vi "CSM Batch Format Tool.vi"() -> ()   [LabVIEW 2017]
doc: "Switch the language of CSM module VI descriptions and comments. Currently supports Chinese and English."
uses:
  <vilib>/Utility/miscctls.llb/LVRectTypeDef.ctl
  _csmHelper/Utility/Is CSM Module - VIRef.vi
  _csmHelper/API/Create From Basic Refs.vi
  _csmHelper/API/Save Instrument.vi
  _csmHelper/API/Destroy.vi
  _csmDoc/csmdoc.lvlib
  Communicable State Machine.lvlib
  _csmHelper/Utility/CSM-Helper Utility.lvlib
  _csmHelper/CSM-Helper.lvclass
  _csmHelper/API/Open Front Panel.vi
panel:
  in  "Open":bool
  in  "CSM Only?":bool
  in  "Terminate":bool
  in  "Refresh":bool
  in  "Macro: Update VI Title":bool
  in  "Macro: Relocate VI Window":bool
  in  "Macro: Rename Year of copyright":bool
  out "Listbox":i32(listbox)
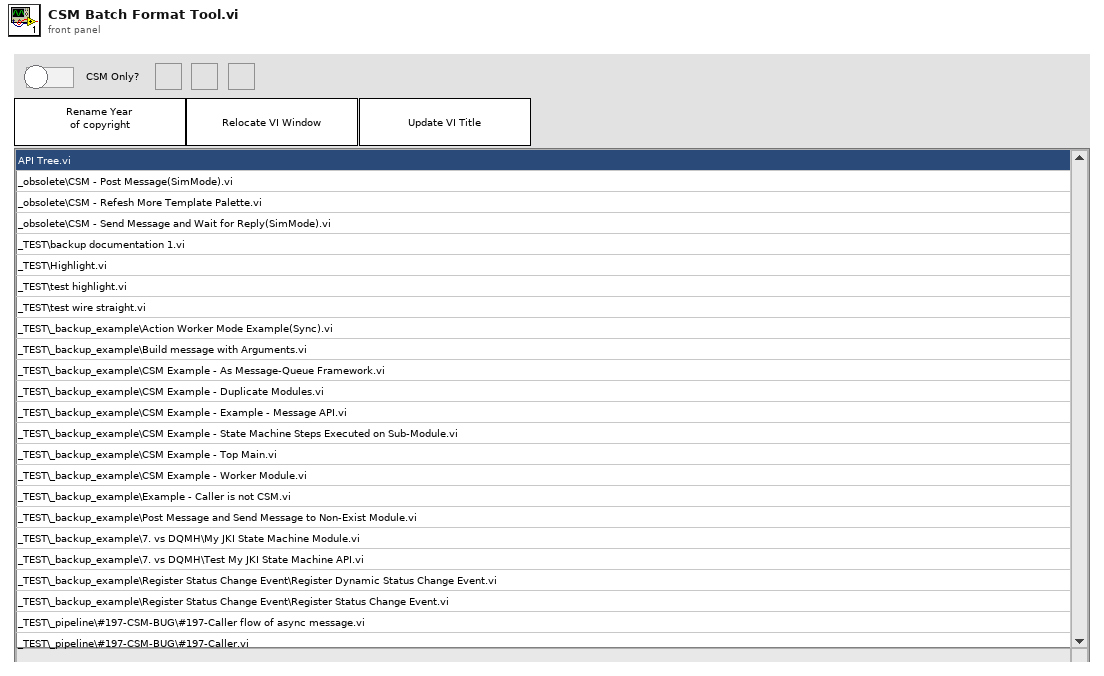
[diagram p1: front panel]
types:
  T1 = enum32{"Invalid", "Standard", "Closed", "Hidden", "Minimized", "Maximized"}
  T2 = enum32{"invalid app kind", "Development System", "Run Time System", "Student Edition", "Embedded LabVIEW", "Evaluation", "Custom"}
  T3 = cluster{"Core":cluster{"Current VI Reference":refnum<vi>, "Close Panel on Exit?":bool}, "VIs":path[], "Success":bool, "Root":path}
  T4 = cluster{"Current VI Reference":refnum<vi>, "Close Panel on Exit?":bool}
  T5 = typedef "CSM-Helper Utility.lvlib/CSM Basic Refs.ctl" = cluster{"VI":refnum<vi>, "While Loop":refnum<vi>, "Case Structure":refnum<vi>, "Parse State Queue":refnum<vi>, "Event Structure":refnum<vi>, "Type":T6}
  T6 = typedef "CSM-Helper Utility.lvlib/CSM Module Type.ctl" = enum16{"Not a CSM", "JKISM", "CSM"}
  T7 = typedef "LVRectTypeDef.ctl" = cluster{"Left":i16, "Top":i16, "Right":i16, "Bottom":i16}
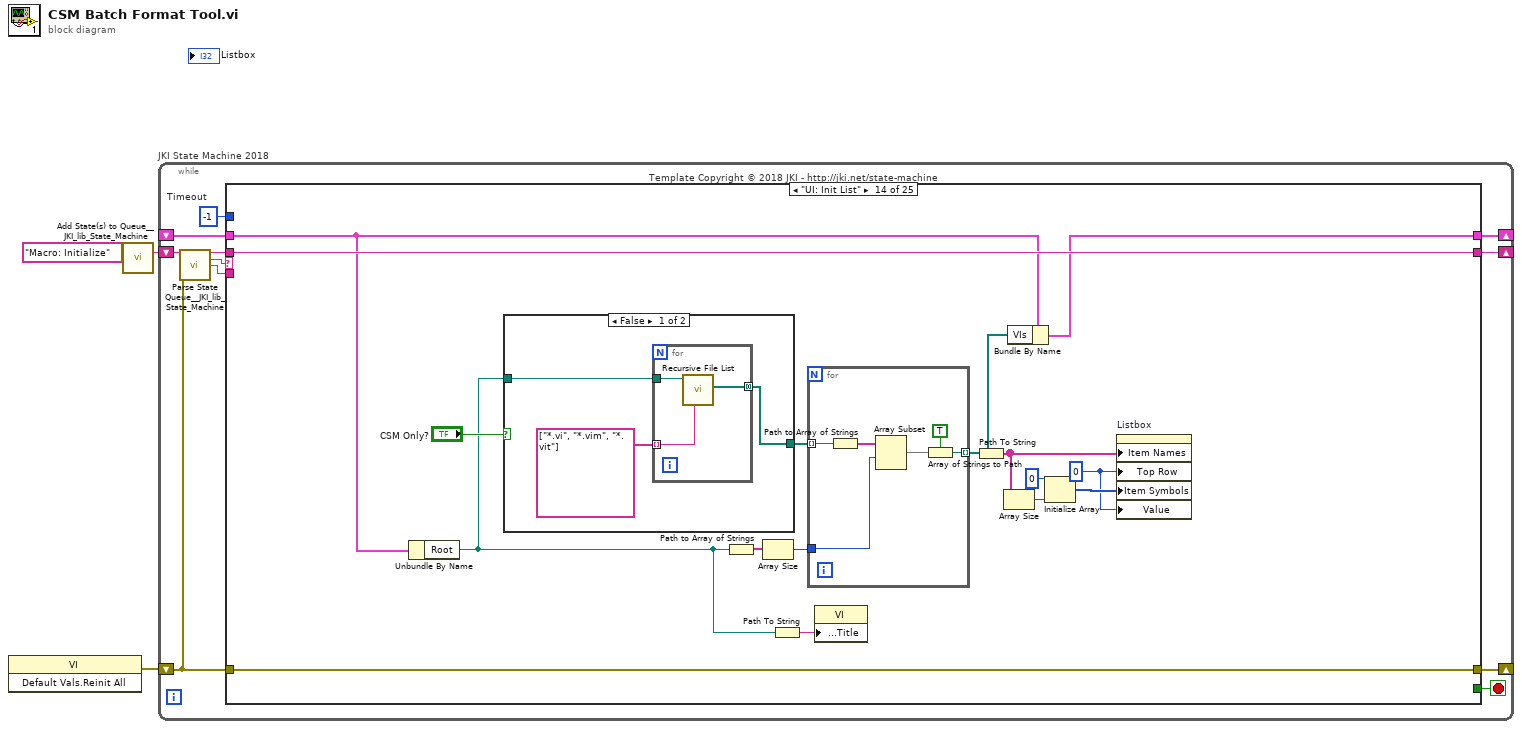
[diagram p0: block diagram]
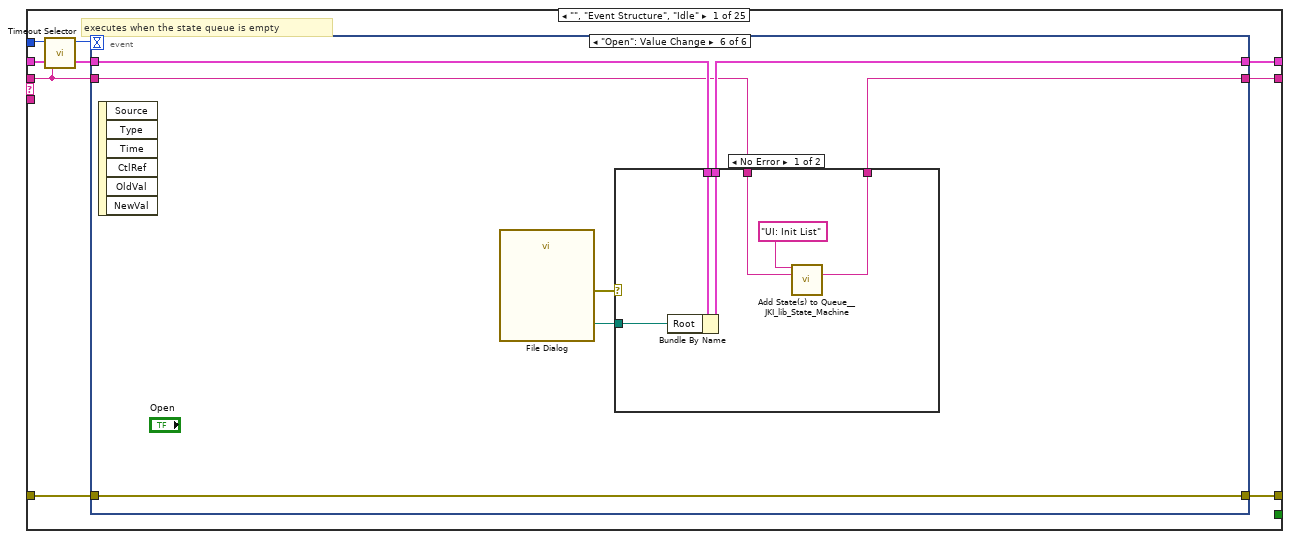
[diagram p2: hidden frame]
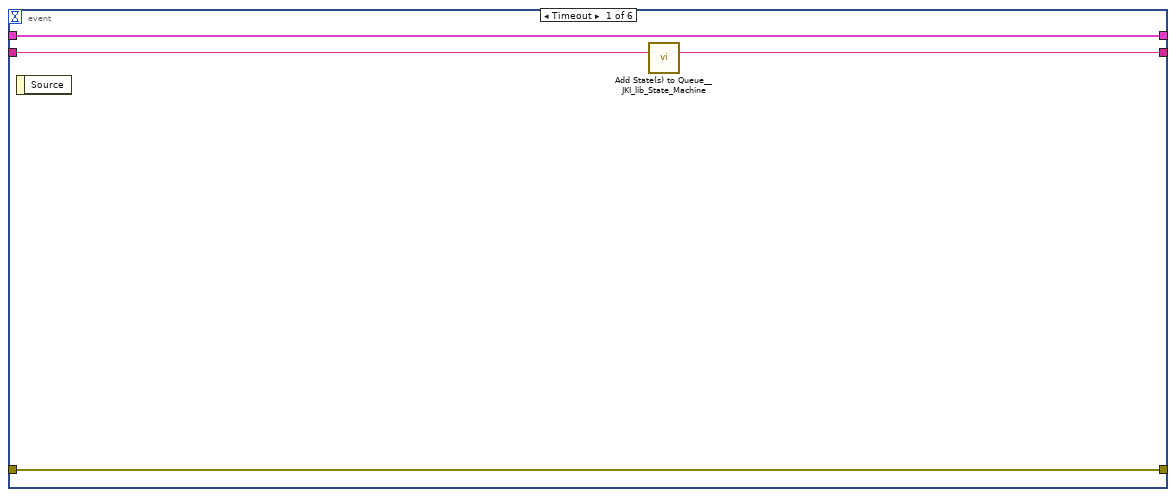
[diagram p3: hidden frame]
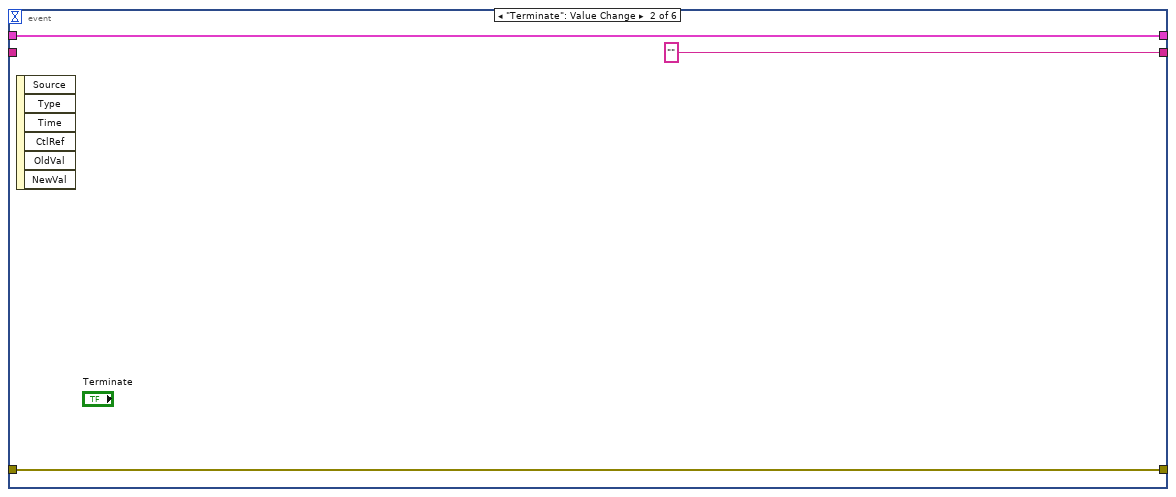
[diagram p4: hidden frame]
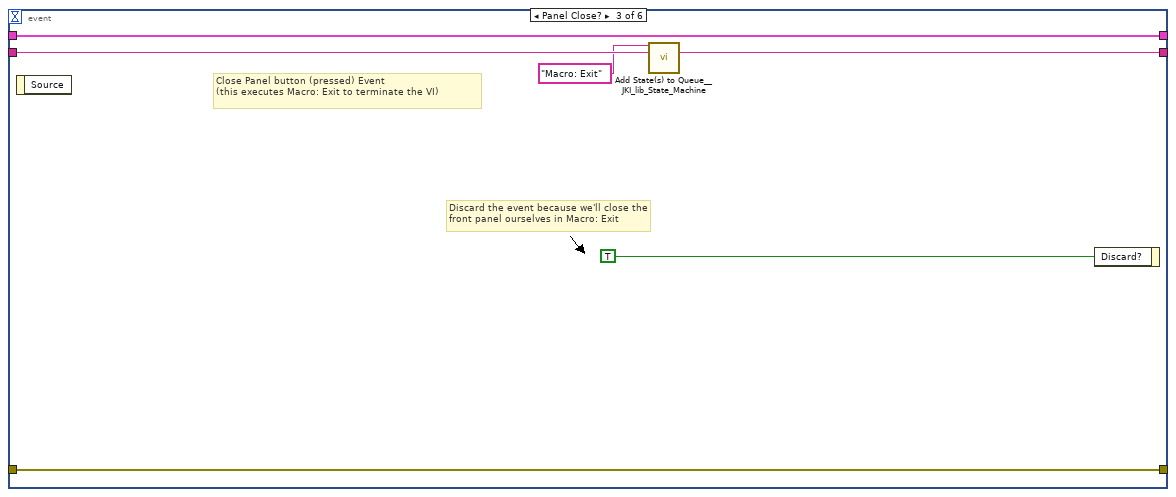
[diagram p5: hidden frame]
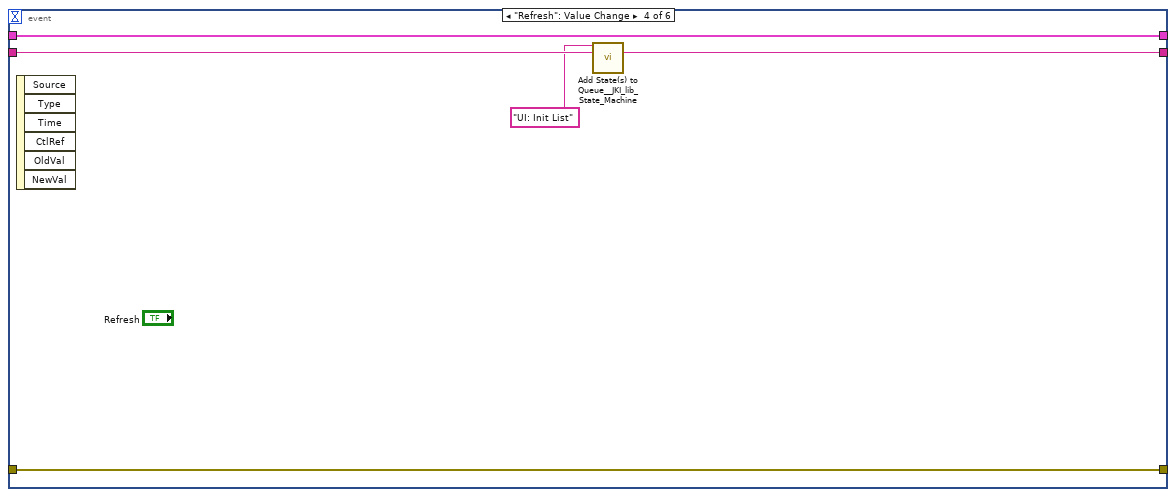
[diagram p6: hidden frame]
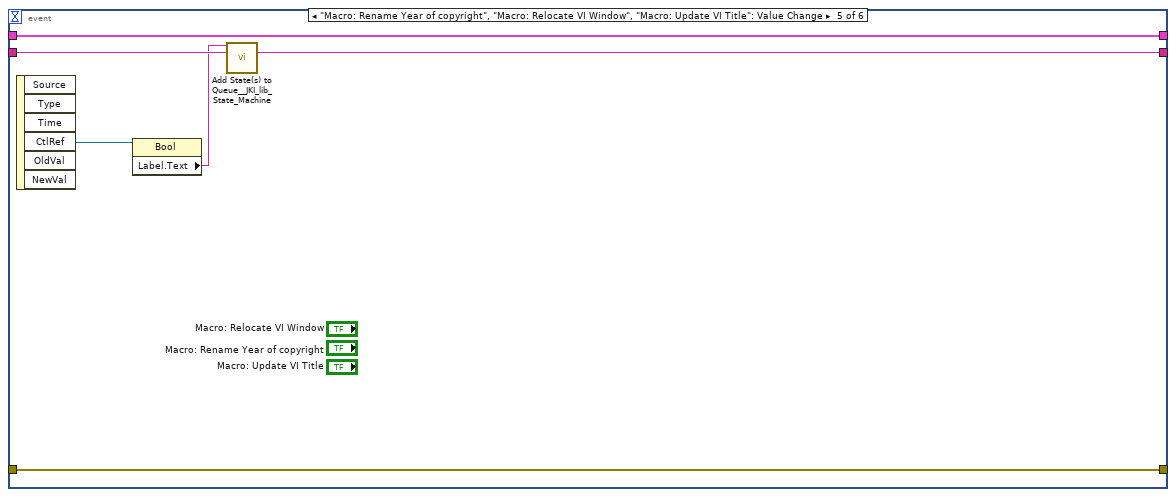
[diagram p7: hidden frame]
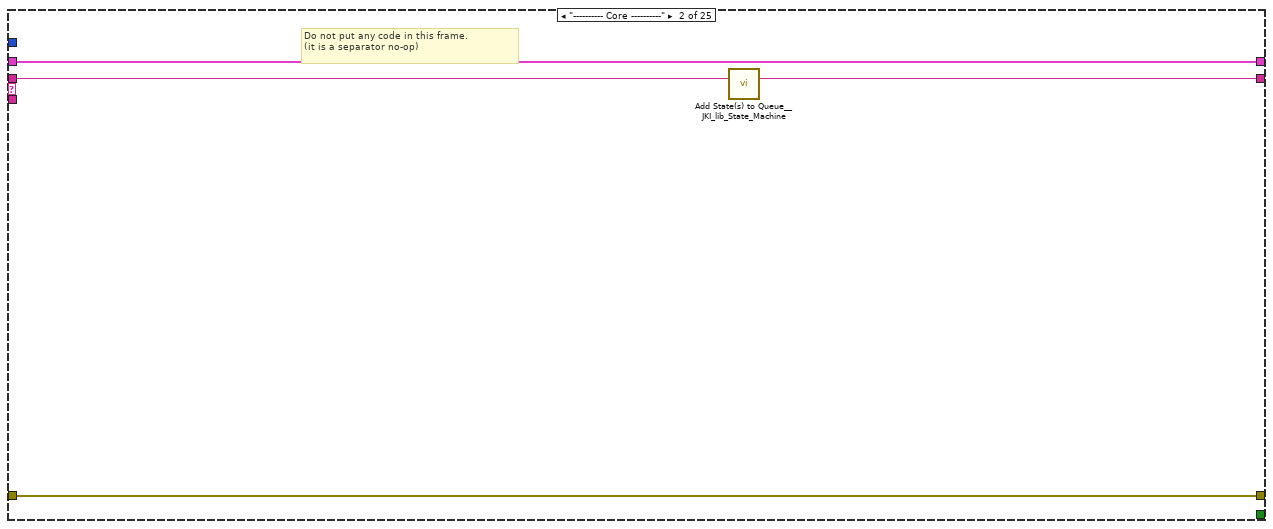
[diagram p9: hidden frame]
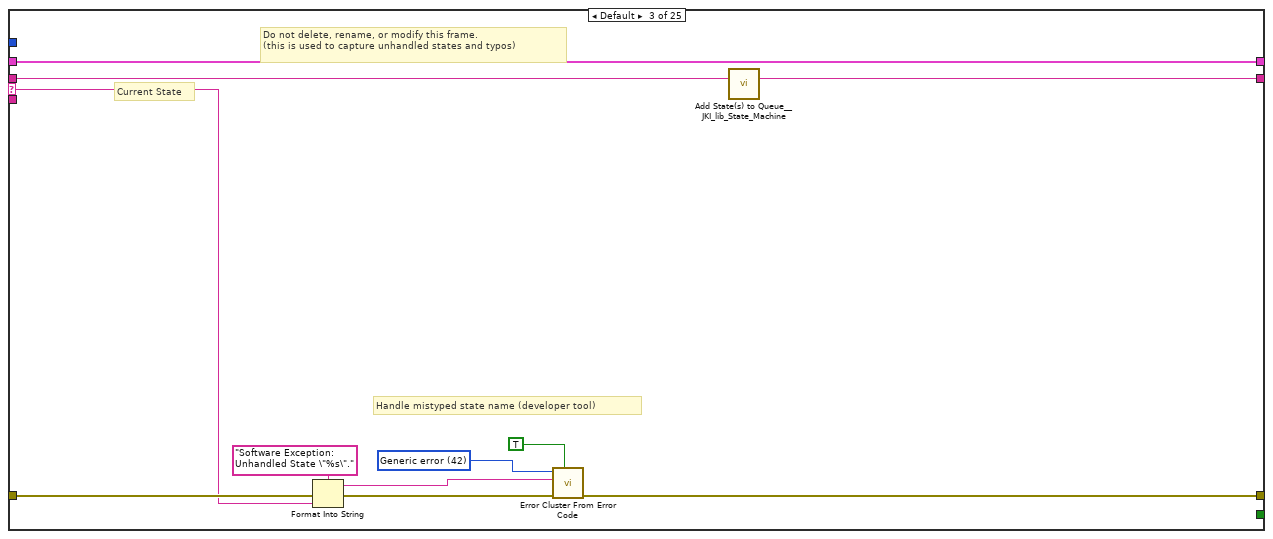
[diagram p10: hidden frame]
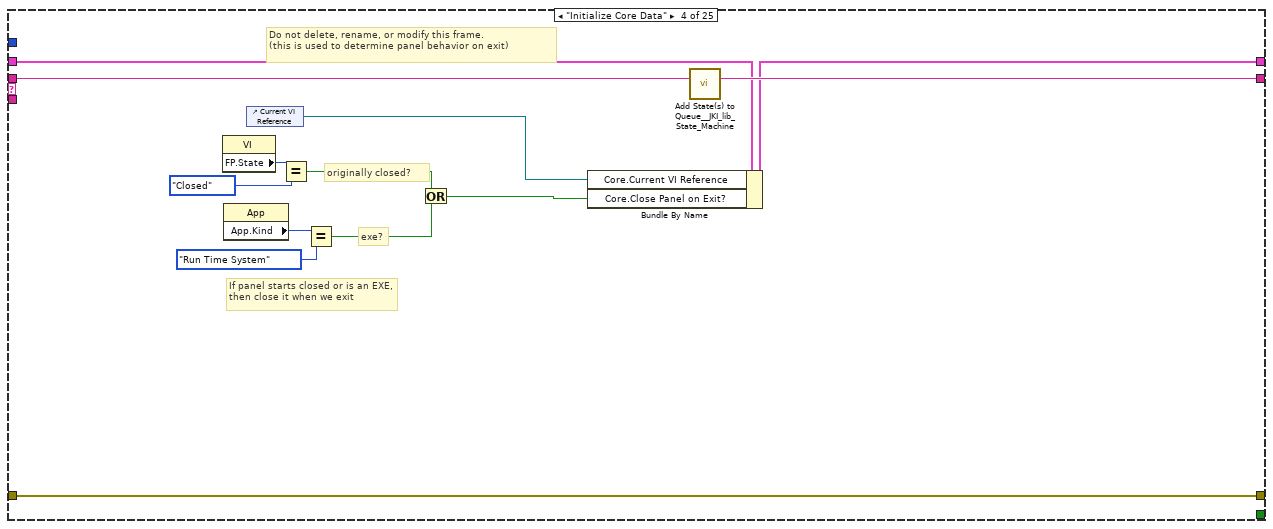
[diagram p11: hidden frame]
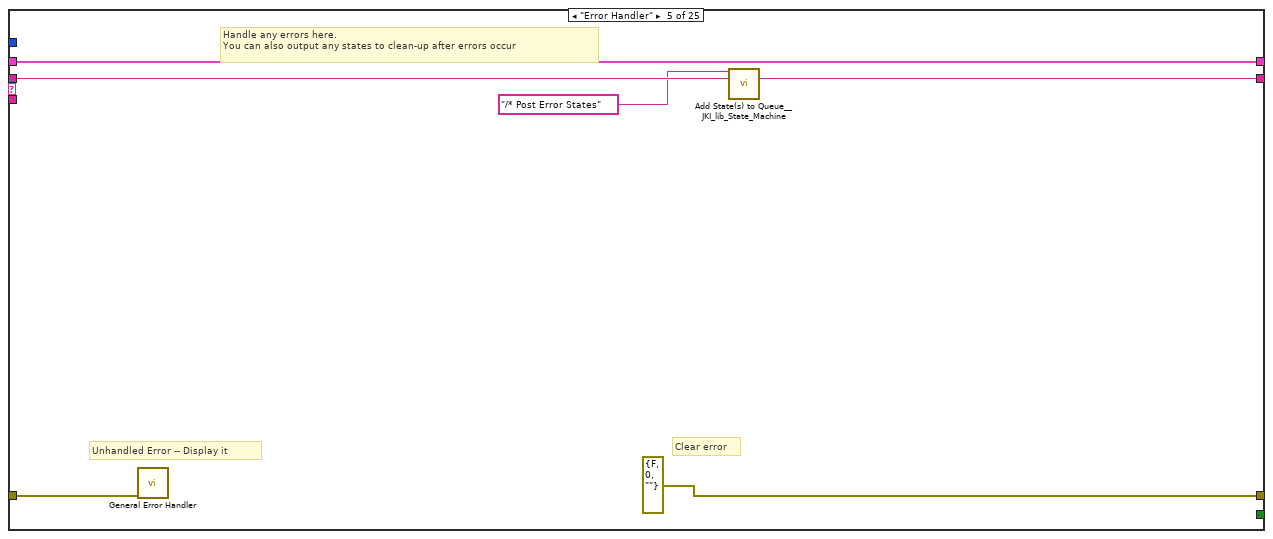
[diagram p12: hidden frame]
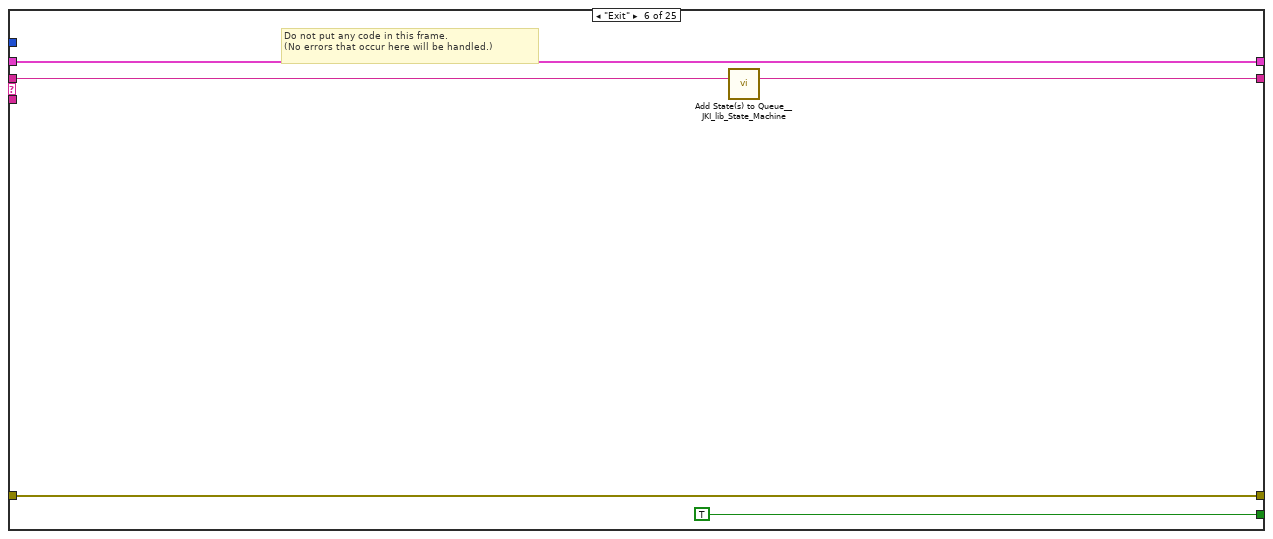
[diagram p13: hidden frame]
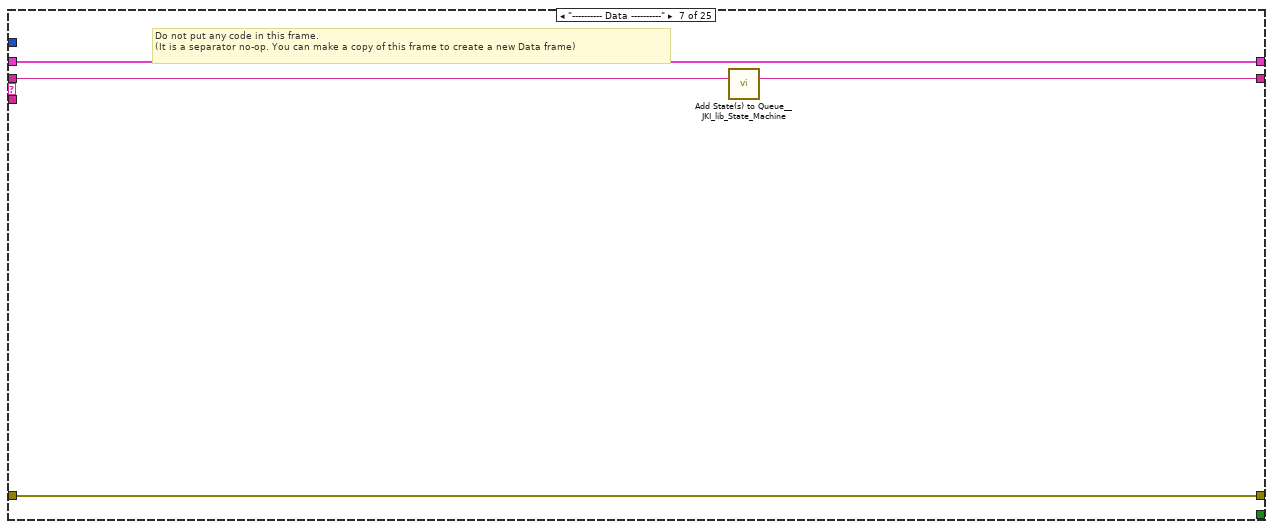
[diagram p14: hidden frame]
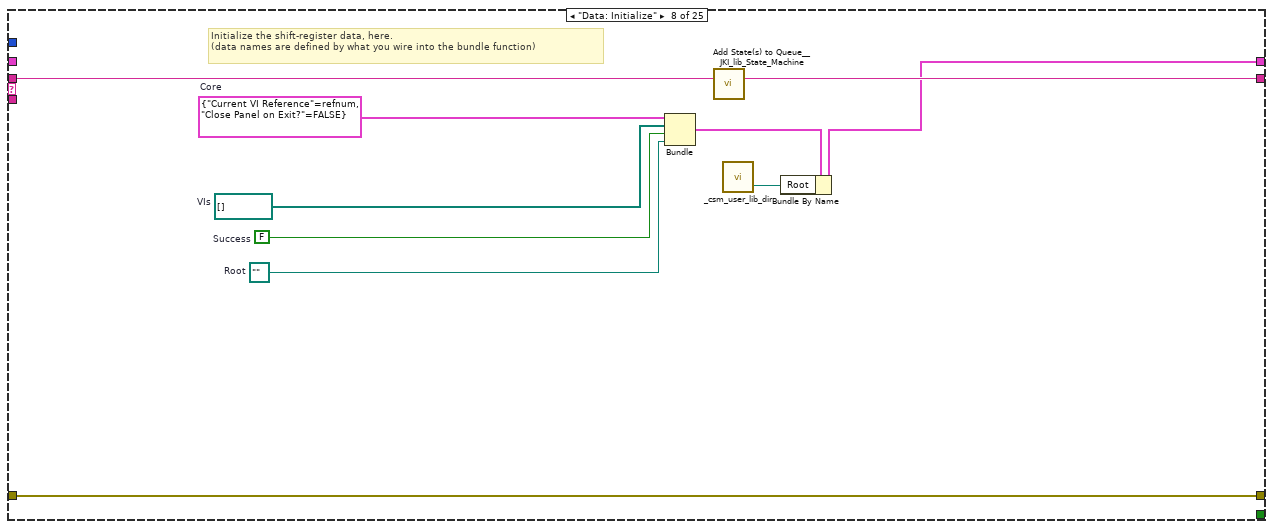
[diagram p15: hidden frame]
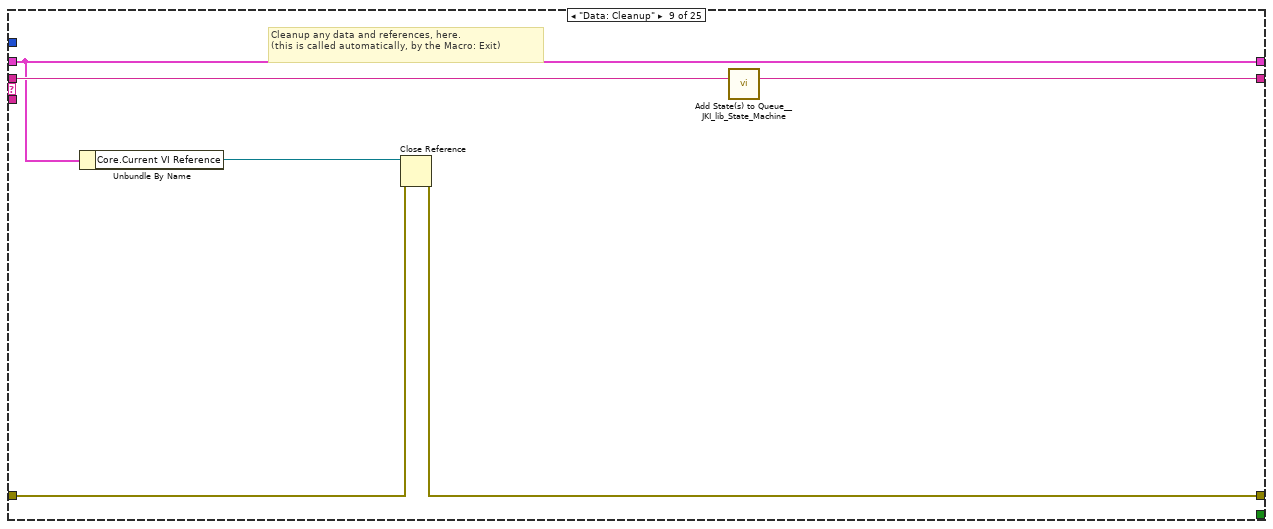
[diagram p16: hidden frame]
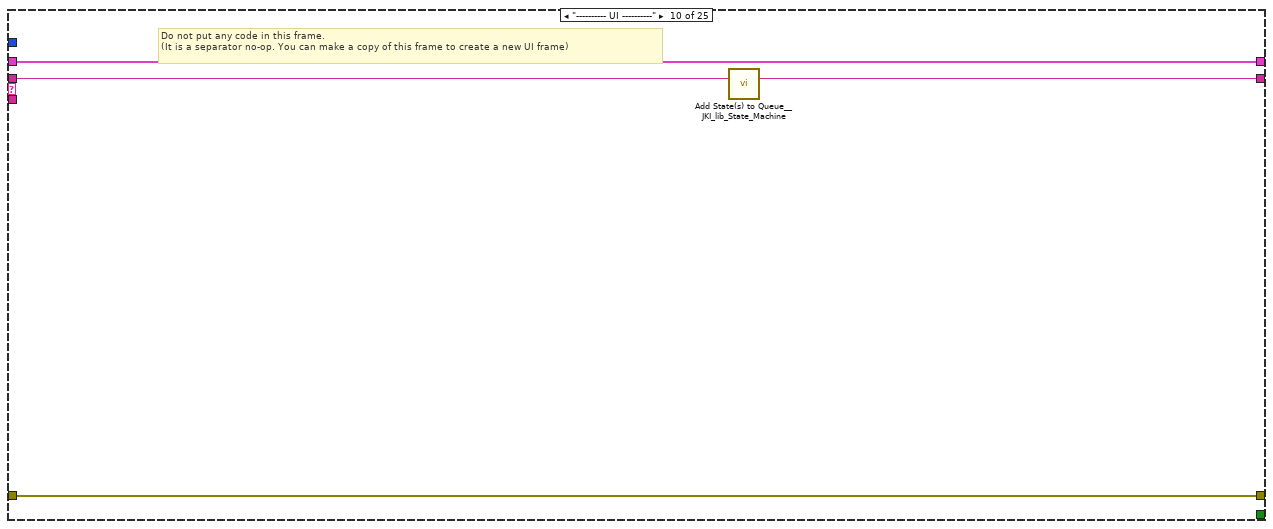
[diagram p17: hidden frame]
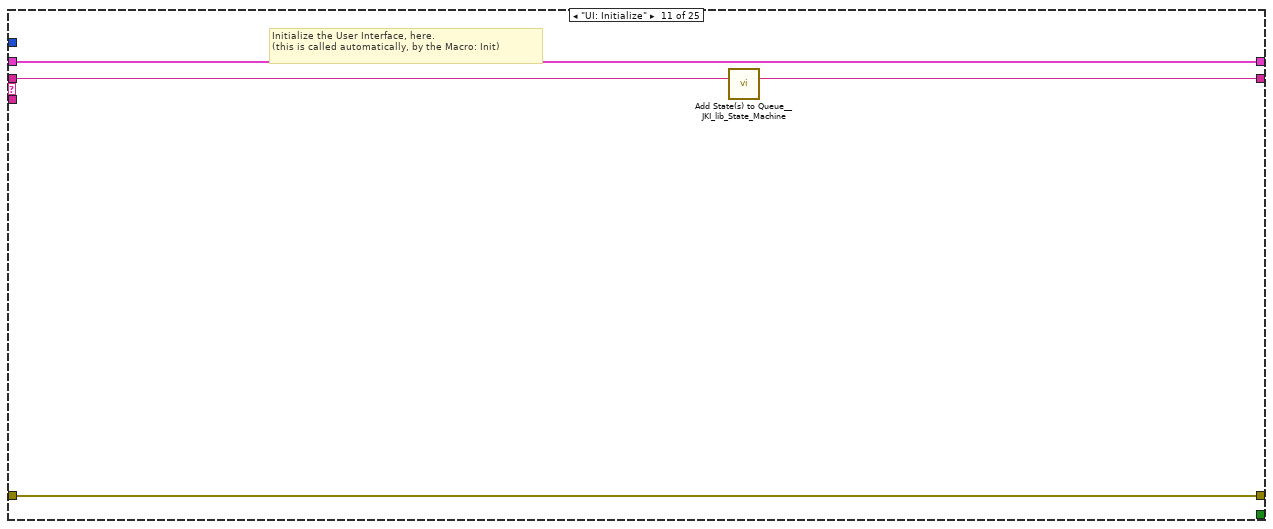
[diagram p18: hidden frame]
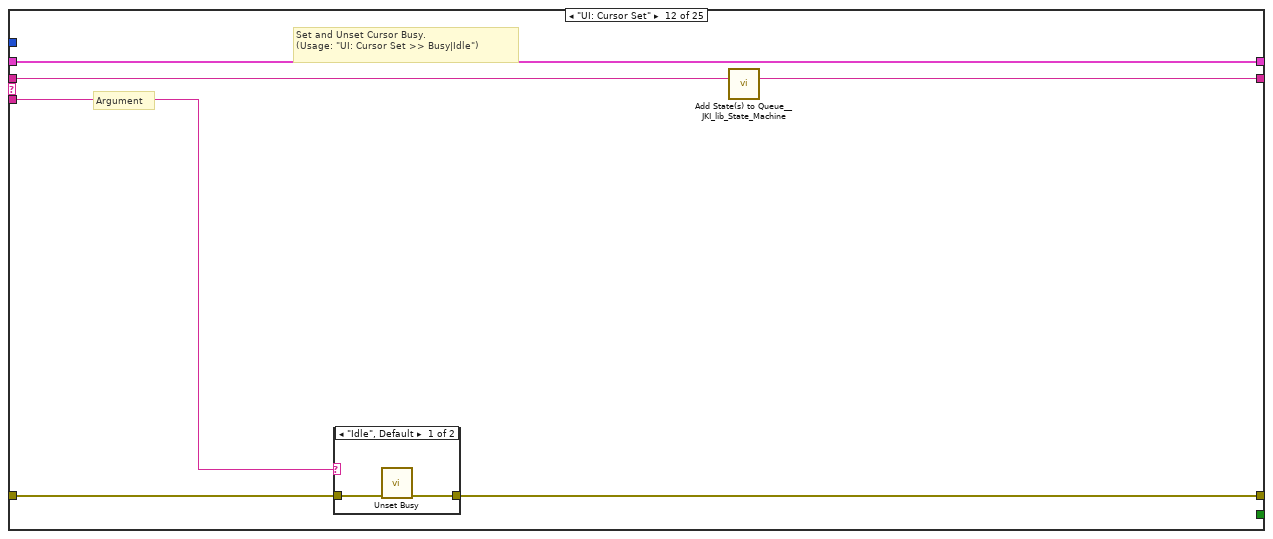
[diagram p19: hidden frame]
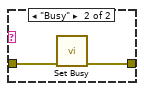
[diagram p20: hidden frame]
diagram:
  n1 = invoke class="VI" method="Default Vals.Reinit All"() -> (error out=w1:errorcluster)  [unwired: 3 in, 2 out]
  n2 = call <vilib>:"Add State(s) to Queue__JKI_lib_State_Machine.vi"("State(s) in (\"\")"="Macro: Initialize") -> ("States Out"=w3:string)  [unwired: 14 in]
  n3 = while "JKI State Machine 2018" {
    shift-right: [w7] -> _
    shift-left: _ -> [w6]
    shift-right: [w10] -> _
    shift-left: w1 -> [w4]
    shift-right: [w9] -> _
    shift-left: w3 -> [w11]
    stop <- w8 stop-if-true
    w5 = -1  # Timeout
    # "Template Copyright © 2018 JKI - http://jki.net/state-machine"
    n4 = call <vilib>:"Parse State Queue__JKI_lib_State_Machine.vi"("State Queue"=w11, "Error In (no error)"=w4) -> ("Remaining States"=w13:string, "Current State"=w14:string, "Arguments"=w12:string)  [unwired: 11 in]
    n5 = case shown="\"UI: Init List\"" w14 {
      selector: w14 -> [_ _ w66 _ _ _ _ _ _ _ _ _ _ _ _ _ _ _ _ _ _ _ _ _ _]
      tunnel: w13 -> [w17 w65 w70 w89 w95 w100 w104 w114 w120 w124 w128 w134 w145 w225 w249 w273 w278 w288 w292 w300 w311 w322 w330 w402 w448]
      tunnel: w12 -> [_ _ _ _ _ _ _ _ _ _ _ w129 w139 _ _ _ _ _ _ _ _ _ w338 w407 w445]
      tunnel: w6 -> [w21 w62 w68 w82 w92 w98 w101 _ w115 w121 w125 w132 w141 w213 w255 w270 w275 w285 w289 w297 w308 w319 w326 w372 w438]
      tunnel: [w20 w63 w72 w86 errorcluster {"status"=FALSE, "code"=0, "source"=""} ("error out") w97 w102 w111 w116 w122 w126 w130 w142 w226 w269 w271 w276 w286 w290 w298 w309 w320 _ _ _] -> w10
      tunnel: w4 -> [w19 w63 w71 w86 w91 w97 w102 w111 w117 w122 w126 w131 w143 w226 w269 w271 w276 w286 w290 w298 w309 w320 _ _ _]
      tunnel: [w22 w64 w69 w88 w94 w99 w103 w113 w119 w123 w127 w133 w144 w225 w250 w272 w277 w287 w291 w299 w310 w321 w331 w403 w449] -> w9
      tunnel: [_ _ _ _ _ TRUE _ _ _ _ _ _ _ _ _ _ _ _ _ _ _ _ _ _ _] -> w8
      tunnel: [w18 w62 w68 w87 w92 w98 w101 w106 w115 w121 w125 w132 w141 w215 w257 w270 w275 w285 w289 w297 w308 w319 w334 w406 w442] -> w7
      tunnel: w5 -> [w16 _ _ _ _ _ _ _ _ _ _ _ _ _ _ _ _ _ _ _ _ _ _ _ _]
      frame "", "Event Structure", "Idle" {
        # "executes when the state queue is empty"
        n6 = call "Timeout Selector.vi"("Remaining States"=w17, "Timeout Expected"=w16) -> ("Timeout"=w15:i32)  [unwired: 5 in]
        n7 = event shown="[5] \"Open\": Value Change" {
          selector: _ -> [_ _ _ _ _ _]
          dyn-events: _ -> [_ _ _ _ _ _]
          timeout: w15 -> [_ _ _ _ _ _]
          tunnel: w17 -> [w26 _ w35 w37 w43 w48]
          tunnel: [w25 "" ("States Out") w34 w38 w44 w49] -> w22
          tunnel: w21 -> [w23 w28 w32 w39 w45 w52]
          tunnel: [w24 w29 w33 w40 w46 w53] -> w20
          tunnel: w19 -> [w24 w29 w33 w40 w46 w53]
          tunnel: [w23 w28 w32 w39 w45 w51] -> w18
          event Timeout {
            n8 = event-data() -> ()  [unwired: 1 in, 1 out]
            n9 = call <vilib>:"Add State(s) to Queue__JKI_lib_State_Machine.vi"("State(s) in (\"\")"=w26) -> ("States Out"=w25:string)  [unwired: 14 in]
          }
          event "Terminate": Value Change {
            n10 = event-data() -> ()  [unwired: 1 in, 6 out]
          }
          event Panel Close? {
            # "Discard the event because we'll close the front panel ourselves in Macro: Exit"
            # "Close Panel button (pressed) Event\n(this executes Macro: Exit to terminate the VI)"
            n11 = event-data() -> ()  [unwired: 1 in, 1 out]
            n12 = call <vilib>:"Add State(s) to Queue__JKI_lib_State_Machine.vi"("State(s) in Front (\"\")"="Macro: Exit", "State(s) in (\"\")"=w35) -> ("States Out"=w34:string)  [unwired: 13 in]
            n13 = event-data("Discard?"=TRUE) -> ()  [unwired: 1 in, 1 out]
          }
          event "Refresh": Value Change {
            n14 = event-data() -> ()  [unwired: 1 in, 6 out]
            n15 = call <vilib>:"Add State(s) to Queue__JKI_lib_State_Machine.vi"("State(s) in Front (\"\")"="UI: Init List" ("State(s) in Front (\"\")"), "State(s) in (\"\")"=w37) -> ("States Out"=w38:string)  [unwired: 13 in]
          }
          event "Macro: Rename Year of copyright", "Macro: Relocate VI Window", "Macro: Update VI Title": Value Change {
            n16 = event-data() -> ("CtlRef"=w42:refnum<vi>)  [unwired: 1 in, 5 out]
            n17 = property class="Bool"(reference=w42) -> ("Label.Text"=w41:string)  [unwired: 1 in, 2 out]
            n18 = call <vilib>:"Add State(s) to Queue__JKI_lib_State_Machine.vi"("State(s) in Front (\"\")"=w41, "State(s) in (\"\")"=w43) -> ("States Out"=w44:string)  [unwired: 13 in]
          }
          event "Open": Value Change {
            n19 = event-data() -> ()  [unwired: 1 in, 6 out]
            n20 = call "File Dialog"() -> ("selected path"=w50:path, "error out"=w47:errorcluster)  [unwired: 12 in, 2 out]
            n21 = case shown="No Error" w47 {
              tunnel: w52 -> [w59 w61]
              tunnel: [w58 w61] -> w51
              tunnel: w50 -> [w57 _]
              tunnel: [w56 w60] -> w49
              tunnel: w48 -> [w55 w60]
              frame No Error {
                n22 = Bundle By Name(cluster=w59, "Root"=w57) -> (w58:T3)
                n23 = call <vilib>:"Add State(s) to Queue__JKI_lib_State_Machine.vi"("State(s) in Front (\"\")"="UI: Init List" ("State(s) in Front (\"\")"), "State(s) in (\"\")"=w55) -> ("States Out"=w56:string)  [unwired: 13 in]
              }
              frame Error {
              }
            }
          }
        }
      }
      frame "---------- Core ----------" {
        # "Do not put any code in this frame.\n(it is a separator no-op)"
        n24 = call <vilib>:"Add State(s) to Queue__JKI_lib_State_Machine.vi"("State(s) in (\"\")"=w65) -> ("States Out"=w64:string)  [unwired: 14 in]
      }
      frame Default {
        w75 = 42 items=["No error", "Argument error", "Memory is full", "Out of zone", "End of file", "File already open", "Generic file I/O error", "File not found", "File permission error", "Disk is full", "Duplicate path", "Too many files open", "System feature not enabled", "Resource file not found", "Cannot add resource", "Resource not found", "Image not found", "Image memory error", "Pen does not exist", "Config type invalid", "Config token not found", "Config parse error", "Config memory error", "Bad external code format", "Bad external code offset", "External code not present", "Null window", "Destroy window error", "Null menu", "Print aborted", "Bad print record", "Print driver error", "Windows error during printing", "Memory error during printing", "Print dialog error", "Generic print error", "Invalid device refnum", "Device not found", "Device parameter error", "Device unit error", "Cannot open device", "Device call aborted", "Generic error", "Cancelled by user", "Object ID too low", "Object ID too high", "Object not in heap", "Unknown heap", "Unknown object (invalid DefProc)", "Unknown object (DefProc not in table)", "Message out of range", "Invalid (null) method", "Unknown message", "Manager call not supported", "Bad address", "Network operation in progress", "Network operation timed out", "Connection is busy", "Network attribute not supported", "Network error", "Address in use", "System out of memory", "Connection aborted", "Connection refused", "Not connected", "Already connected", "Connection closed", "Initialization error (interapplication manager)", "Bad occurrence", "Wait on unbound occurrence handler", "Occurrence queue overflow", "Datalog type conflict", "Unused", "Unrecognized type (interapplication manager)", "Memory corrupt", "Failed to make temporary DLL", "Old CIN version", "Drag socket not found", "Failed to load drop-object", "Failed to register OLE object", "Failed to release OLE object", "Format specifier type mismatch", "Unknown format specifier", "Too few format specifiers", "Too many format specifiers", "Scan failed", "Newer CIN version", "Error converting to variant", "Runtime menu error", "Password tampered", "Variant attribute not found", "Incompatible variant data type", "Event data is not available", "Event Store is not present", "Occurrence is not found", "Event Queue is not created", "Event info is not available", "Refnum passed is NULL", "Error retrieving Class GUID", "Error retrieving CoClass GUID", "Error retrieving TypeLib GUID.", "Bad built application magic bytes.", "Specific driver is different from the specific driver associated with the Logical Name.", "There is no session opened to the class driver.", "Max Error", "MAX - Error with config objects", "MAX - Error loading configuration", "MAX - Group not supported"]
        # "Current State"
        # "Do not delete, rename, or modify this frame.\n(this is used to capture unhandled states and typos)"
        # "Handle mistyped state name (developer tool)"
        n25 = Format Into String(format string="Software Exception: Unhandled State \"%s\"." ("message"), error in=w71, w66) -> (resulting string=w74:string, error out=w73:errorcluster)  [unwired: 1 in]
        n26 = call <vilib>:"Error Cluster From Error Code.vi"("show call chain? (False)"=TRUE, "error in (no error)"=w73, "error message (\"\")"=w74, "error code (0)"=w75) -> ("error out"=w72:errorcluster)  [unwired: 5 in]
        n27 = call <vilib>:"Add State(s) to Queue__JKI_lib_State_Machine.vi"("State(s) in (\"\")"=w70) -> ("States Out"=w69:string)  [unwired: 14 in]
      }
      frame "Initialize Core Data" {
        # "Do not delete, rename, or modify this frame.\n(this is used to determine panel behavior on exit)"
        # "originally closed?"
        # "exe?"
        # "If panel starts closed or is an EXE, then close it when we exit"
        n28 = property class="VI"() -> ("FP.State"=w79:T1)  [unwired: 2 in, 2 out]
        n29 = property class="App"() -> ("App.Kind"=w85:T2)  [unwired: 2 in, 2 out]
        n30 = control-ref of="Current VI Reference"() -> (w80:refnum<vi>)
        n31 = Equal?(x=w79, y=T1."Closed" ("Front Panel Window:State")) -> (x = y?=w77:bool)
        n32 = Equal?(x=w85, y=T2."Run Time System" ("Application:Kind")) -> (x = y?=w83:bool)
        n33 = Or(x=w77, y=w83) -> (x .or. y?=w81:bool)
        n34 = Bundle By Name(cluster=w82, "Core.Current VI Reference"=w80, "Core.Close Panel on Exit?"=w81) -> (w87:T3)
        n35 = call <vilib>:"Add State(s) to Queue__JKI_lib_State_Machine.vi"("State(s) in (\"\")"=w89) -> ("States Out"=w88:string)  [unwired: 14 in]
      }
      frame "Error Handler" {
        # "Unhandled Error -- Display it"
        # "Handle any errors here.\nYou can also output any states to clean-up after errors occur"
        # "Clear error"
        n36 = call <vilib>:"General Error Handler.vi"("error in (no error)"=w91) -> ()  [unwired: 10 in, 5 out]
        n37 = call <vilib>:"Add State(s) to Queue__JKI_lib_State_Machine.vi"("State(s) in Front (\"\")"="/* Post Error States", "State(s) in (\"\")"=w95) -> ("States Out"=w94:string)  [unwired: 13 in]
      }
      frame "Exit" {
        # "Do not put any code in this frame.\n(No errors that occur here will be handled.)"
        n38 = call <vilib>:"Add State(s) to Queue__JKI_lib_State_Machine.vi"("State(s) in (\"\")"=w100) -> ("States Out"=w99:string)  [unwired: 14 in]
      }
      frame "---------- Data ----------" {
        # "Do not put any code in this frame.\n(It is a separator no-op. You can make a copy of this frame to create a new Data frame)"
        n39 = call <vilib>:"Add State(s) to Queue__JKI_lib_State_Machine.vi"("State(s) in (\"\")"=w104) -> ("States Out"=w103:string)  [unwired: 14 in]
      }
      frame "Data: Initialize" {
        w107 = path ""  # Root
        w108 = FALSE  # Success
        w109 = path[] []  # VIs
        w110 = T4 {"Current VI Reference"=refnum, "Close Panel on Exit?"=FALSE}  # Core
        # "Initialize the shift-register data, here.\n(data names are defined by what you wire into the bundle function)"
        n40 = Bundle("Core"=w110, "VIs"=w109, "Success"=w108, "Root"=w107) -> (w112:T3)  [unwired: 1 in]
        n41 = call <vilib>:"Add State(s) to Queue__JKI_lib_State_Machine.vi"("State(s) in (\"\")"=w114) -> ("States Out"=w113:string)  [unwired: 14 in]
        n42 = call "_csm_user_lib_dir.vi"() -> ("<LabVIEW>"=w105:path)  [unwired: 2 in, 1 out]
        n43 = Bundle By Name(cluster=w112, "Root"=w105) -> (w106:T3)
      }
      frame "Data: Cleanup" {
        # "Cleanup any data and references, here.\n(this is called automatically, by the Macro: Exit)"
        n44 = Unbundle By Name(w115) -> ("Core.Current VI Reference"=w118:refnum<vi>)
        n45 = Close Reference(reference=w118, error in (no error)=w117) -> (error out=w116:errorcluster)
        n46 = call <vilib>:"Add State(s) to Queue__JKI_lib_State_Machine.vi"("State(s) in (\"\")"=w120) -> ("States Out"=w119:string)  [unwired: 14 in]
      }
      frame "---------- UI ----------" {
        # "Do not put any code in this frame.\n(It is a separator no-op. You can make a copy of this frame to create a new UI frame)"
        n47 = call <vilib>:"Add State(s) to Queue__JKI_lib_State_Machine.vi"("State(s) in (\"\")"=w124) -> ("States Out"=w123:string)  [unwired: 14 in]
      }
      frame "UI: Initialize" {
        # "Initialize the User Interface, here.\n(this is called automatically, by the Macro: Init)"
        n48 = call <vilib>:"Add State(s) to Queue__JKI_lib_State_Machine.vi"("State(s) in (\"\")"=w128) -> ("States Out"=w127:string)  [unwired: 14 in]
      }
      frame "UI: Cursor Set" {
        # "Argument"
        # "Set and Unset Cursor Busy.\n(Usage: \"UI: Cursor Set >> Busy|Idle\")"
        n49 = case shown="\"Idle\", Default" w129 {
          tunnel: w131 -> [w136 w138]
          tunnel: [w135 w137] -> w130
          frame "Idle", Default {
            n50 = call <vilib>:"Unset Busy.vi"("error in (no error)"=w136) -> ("error out"=w135:errorcluster)  [unwired: 10 in]
          }
          frame "Busy" {
            n51 = call <vilib>:"Set Busy.vi"("error in (no error)"=w138) -> ("error out"=w137:errorcluster)  [unwired: 9 in, 1 out]
          }
        }
        n52 = call <vilib>:"Add State(s) to Queue__JKI_lib_State_Machine.vi"("State(s) in (\"\")"=w134) -> ("States Out"=w133:string)  [unwired: 14 in]
      }
      frame "UI: Front Panel State" {
        # "Argument"
        # "Set Front Panel Open or Closed\n(Usage: \"UI: Front Panel State >> Open|Close\")"
        n53 = Unbundle By Name(w141) -> ("Core.Current VI Reference"=w140:refnum<vi>)
        n54 = case shown="\"Minimize\", \"Minimized\"" w139 {
          tunnel: w143 -> [w151 w166 w177 w190 w203]
          tunnel: [w153 w167 w179 w192 w205] -> w142
          tunnel: w140 -> [w152 w164 w178 w191 w204]
          frame "Open", "Standard", Default {
            w146 = T1."Standard" ("State")
            n55 = property class="VI"(reference=w152, error in=w151) -> (reference out=w149:refnum<vi>, error out=w150:errorcluster, "FP.State"=w148:T1)
            n56 = Not Equal?(x=w148, y=w146) -> (x != y?=w147:bool)
            n57 = case shown="True" w147 {
              tunnel: [w157 w159] -> w153
              tunnel: w150 -> [w156 w159]
              tunnel: w149 -> [w155 _]
              tunnel: w146 -> [w154 _]
              frame True {
                n58 = invoke class="VI" method="FP.Open"(reference=w155, error in=w156, "Activate"=TRUE, "State"=w154) -> (error out=w157:errorcluster)  [unwired: 1 in, 4 out]
              }
              frame False {
              }
            }
          }
          frame "Close", "Closed" {
            n59 = property class="VI"(reference=w164, error in=w166) -> (reference out=w163:refnum<vi>, error out=w165:errorcluster, "FP.State"=w161:T1)
            n60 = Not Equal?(x=w161, y=T1."Closed" ("Front Panel Window:State")) -> (x != y?=w160:bool)
            n61 = case shown="True" w160 {
              tunnel: [w168 w171] -> w167
              tunnel: w165 -> [w168 w170]
              tunnel: w163 -> [_ w169]
              frame False {
              }
              frame True {
                n62 = invoke class="VI" method="FP.Close"(reference=w169, error in=w170) -> (error out=w171:errorcluster)  [unwired: 1 in, 2 out]
              }
            }
          }
          frame "Hidden", "Hide" {
            w172 = T1."Hidden" ("State")
            n63 = property class="VI"(reference=w178, error in=w177) -> (reference out=w175:refnum<vi>, error out=w176:errorcluster, "FP.State"=w174:T1)
            n64 = Not Equal?(x=w174, y=w172) -> (x != y?=w173:bool)
            n65 = case shown="True" w173 {
              tunnel: [w183 w184] -> w179
              tunnel: w176 -> [w182 w184]
              tunnel: w175 -> [w181 _]
              tunnel: w172 -> [w180 _]
              frame True {
                n66 = invoke class="VI" method="FP.Open"(reference=w181, error in=w182, "State"=w180) -> (error out=w183:errorcluster)  [unwired: 2 in, 4 out]
              }
              frame False {
              }
            }
          }
          frame "Minimize", "Minimized" {
            w185 = T1."Minimized" ("State")
            n67 = property class="VI"(reference=w191, error in=w190) -> (reference out=w188:refnum<vi>, error out=w189:errorcluster, "FP.State"=w187:T1)
            n68 = Not Equal?(x=w187, y=w185) -> (x != y?=w186:bool)
            n69 = case shown="True" w186 {
              tunnel: [w196 w197] -> w192
              tunnel: w189 -> [w195 w197]
              tunnel: w188 -> [w194 _]
              tunnel: w185 -> [w193 _]
              frame True {
                n70 = invoke class="VI" method="FP.Open"(reference=w194, error in=w195, "State"=w193) -> (error out=w196:errorcluster)  [unwired: 2 in, 4 out]
              }
              frame False {
              }
            }
          }
          frame "Maximize", "Maximized" {
            w198 = T1."Maximized" ("State")
            n71 = property class="VI"(reference=w204, error in=w203) -> (reference out=w201:refnum<vi>, error out=w202:errorcluster, "FP.State"=w200:T1)
            n72 = Not Equal?(x=w200, y=w198) -> (x != y?=w199:bool)
            n73 = case shown="True" w199 {
              tunnel: [w209 w210] -> w205
              tunnel: w202 -> [w208 w210]
              tunnel: w201 -> [w207 _]
              tunnel: w198 -> [w206 _]
              frame True {
                n74 = invoke class="VI" method="FP.Open"(reference=w207, error in=w208, "State"=w206) -> (error out=w209:errorcluster)  [unwired: 2 in, 4 out]
              }
              frame False {
              }
            }
          }
        }
        n75 = call <vilib>:"Add State(s) to Queue__JKI_lib_State_Machine.vi"("State(s) in (\"\")"=w145) -> ("States Out"=w144:string)  [unwired: 14 in]
      }
      frame "UI: Init List" {
        w220 = 0 ("Top Row")
        n76 = Unbundle By Name(w213) -> ("Root"=w211:path)
        n77 = case shown="False" "CSM Only?" {
          tunnel: [w227 w234] -> w219
          tunnel: w211 -> [w228 _]
          frame False {
            n78 = for {
              tunnel: w228 -> [w232]
              tunnel: string[] ["*.vi", "*.vim", "*.vit"] -> [w231] mode=indexing
              tunnel: [w230] -> w227 mode=concatenating
              n79 = call <vilib>:"Recursive File List.vi"("pattern"=w231, "Folder Path"=w232) -> ("All Files in Dir"=w230:path[])  [unwired: 5 in, 4 out]
            }
          }
          frame True {
            n80 = call "csmdoc_list_all_csm_documented_VIs.vi"("Only CSM Folder"=FALSE) -> ("Array"=w235:path[])  [unwired: 10 in]
            n81 = for {
              tunnel: w235 -> [w239] mode=indexing
              tunnel: [w239] -> w234 mode=indexing if=w238
              n82 = Open VI Reference(vi path=w239, options=2) -> (vi reference=w237:refnum<vi>, error out=w240:errorcluster)  [unwired: 4 in]
              n83 = call-poly "Is CSM Module.vi"("error in (no error)"=w240, "VIRef"=w237) -> ("error out"=w241:errorcluster, "Is CSM Module?"=w238:bool)  [unwired: 7 in, 1 out]
              n84 = Close Reference(reference=w237, error in (no error)=w241) -> ()  [unwired: 1 out]
            }
          }
        }
        n85 = Path to Array of Strings(0:w211) -> (2:w218:string[])  [unwired: 1 out]
        n86 = Array Size(array=w218) -> (size(s)=w217:i32)
        n87 = Path To String(path=w211) -> (string=w212:string)
        n88 = for {
          tunnel: w219 -> [w247] mode=indexing
          tunnel: w217 -> [w245]
          tunnel: [w244] -> w216 mode=indexing
          n89 = Path to Array of Strings(0:w247) -> (2:w246:string[])  [unwired: 1 out]
          n90 = Array Subset(array=w246, index=w245) -> (w243:string[])  [unwired: 1 in]
          n91 = Array of Strings to Path(0:w243, 1:TRUE ("relative")) -> (2:w244:path)
        }
        n92 = property class="VI"("Front Panel.Title"=w212) -> ()  [unwired: 2 in, 2 out]
        n93 = Path To String(path=w216) -> (string=w223:string[])
        n94 = Array Size(array=w223) -> (size(s)=w224:i32)
        n95 = Bundle By Name(cluster=w213, "VIs"=w216) -> (w215:T3)
        n96 = Initialize Array(0 ("Top Row"), w224) -> (w221:i32[])
        n97 = property on="Listbox" class="LstBox (strict)"("Item Names"=w223, "Top Row"=w220, "Item Symbols"=w221, "Value"=w220) -> ()  [unwired: 2 in, 2 out]
      }
      frame "UI: Post Action" {
        n98 = Unbundle By Name(w255) -> ("Success"=w254:bool)
        n99 = control-ref of="Listbox"() -> (w260:refnum<vi>)
        n100 = property on="Property Node" class="LstBox (strict)"(reference=w260) -> (reference out=w259:refnum<vi>, error out=w258:errorcluster, "Value"=w261:i32, "Item Symbols"=w268:i32[])  [unwired: 1 in]
        n101 = Select(t=1 ("new element/subarray"), s=w254, f=2 ("new element/subarray")) -> (s? t:f=w251:i32)
        n102 = Replace Array Subset(array=w268, new element=w251, index=w261) -> (w267:i32[])
        n103 = Subtract(x=w261, y=5) -> (x-y=w264:i32)
        n104 = Increment(x=w261) -> (x+1=w266:i32)
        n105 = Max & Min(x=w264, y=0) -> (max(x,y)=w262:i32)  [unwired: 1 out]
        n106 = property on="Property Node" class="LstBox (strict)"(reference=w259, error in=w258, "Top Row"=w262, "Item Symbols"=w267, "Value"=w266) -> ()  [unwired: 2 out]
        n107 = Bundle By Name(cluster=w255, "Success"=TRUE ("Last Action Success")) -> (w257:T3)
        n108 = call <vilib>:"Add State(s) to Queue__JKI_lib_State_Machine.vi"("State(s) in Front (\"\")"="Idle" ("State(s) in Front (\"\")"), "State(s) in (\"\")"=w249) -> ("States Out"=w250:string)  [unwired: 13 in]
      }
      frame "---------- Macro ----------" {
        # "Do not put any code in this frame.\n(It is a separator no-op. You can make a copy of this frame to create a new Macro frame)"
        n109 = call <vilib>:"Add State(s) to Queue__JKI_lib_State_Machine.vi"("State(s) in (\"\")"=w273) -> ("States Out"=w272:string)  [unwired: 14 in]
      }
      frame "Macro: Initialize" {
        # "Initialization Macro\n(This is called once, when the VI starts)"
        n110 = call <vilib>:"Add State(s) to Queue__JKI_lib_State_Machine.vi"("State(s) in Front (\"\")"="Data: Initialize\nInitialize Core Data\nUI: Initialize\nUI: Front Panel State >> Open\nUI: Init List", "State(s) in (\"\")"=w278) -> ("States Out"=w277:string)  [unwired: 13 in]
      }
      frame "Macro: Exit" {
        # "Exit Macro\n(This is called once, when the VI exits)"
        n111 = Unbundle By Name(w285) -> ("Core.Close Panel on Exit?"=w284:bool)
        n112 = Select(t="UI: Front Panel State >> Close", s=w284, f="") -> (s? t:f=w281:string)
        n113 = call <vilib>:"Add State(s) to Queue__JKI_lib_State_Machine.vi"("State(s) in (\"\")"=w281, "State(s) at Back (\"\")"="Data: Cleanup\nExit") -> ("States Out"=w279:string)  [unwired: 13 in]
        n114 = call <vilib>:"Add State(s) to Queue__JKI_lib_State_Machine.vi"("State(s) in Front (\"\")"=w279, "State(s) in (\"\")"=w288) -> ("States Out"=w287:string)  [unwired: 13 in]
      }
      frame "---------- Action ----------" {
        # "Template Separator\n(You can make a copy of, or modify, this frame)"
        n115 = call <vilib>:"Add State(s) to Queue__JKI_lib_State_Machine.vi"("State(s) in (\"\")"=w292) -> ("States Out"=w291:string)  [unwired: 14 in]
      }
      frame "Macro: Rename Year of copyright" {
        n116 = property on="Listbox" class="LstBox (strict)"() -> ("Item Names"=w296:string[])  [unwired: 2 in, 2 out]
        n117 = for {
          tunnel: w296 -> [w303] mode=indexing
          tunnel: "Action: Rename Year of copyright" ("State") -> [w302]
          tunnel: [w301] -> w294 mode=indexing
          n118 = call <vilib>:"Build State String with Arguments__JKI_lib_State_Machine.vi"("Arguments (\"\")"=w303, "State"=w302) -> ("State with Arguments"=w301:string)  [unwired: 4 in]
        }
        n119 = call "CSM - Compact Multiple States.vi"("Multiple States"=w294) -> ("States"=w293:string)  [unwired: 9 in]
        n120 = call <vilib>:"Add State(s) to Queue__JKI_lib_State_Machine.vi"("State(s) in Front (\"\")"=w293, "State(s) in (\"\")"=w300) -> ("States Out"=w299:string)  [unwired: 13 in]
      }
      frame "Macro: Relocate VI Window" {
        n121 = property on="Listbox" class="LstBox (strict)"() -> ("Item Names"=w307:string[])  [unwired: 2 in, 2 out]
        n122 = for {
          tunnel: w307 -> [w314] mode=indexing
          tunnel: "Action: Relocate VI Window" ("State") -> [w313]
          tunnel: [w312] -> w305 mode=indexing
          n123 = call <vilib>:"Build State String with Arguments__JKI_lib_State_Machine.vi"("Arguments (\"\")"=w314, "State"=w313) -> ("State with Arguments"=w312:string)  [unwired: 4 in]
        }
        n124 = call "CSM - Compact Multiple States.vi"("Multiple States"=w305) -> ("States"=w304:string)  [unwired: 9 in]
        n125 = call <vilib>:"Add State(s) to Queue__JKI_lib_State_Machine.vi"("State(s) in Front (\"\")"=w304, "State(s) in (\"\")"=w311) -> ("States Out"=w310:string)  [unwired: 13 in]
      }
      frame "Macro: Update VI Title" {
        n126 = property on="Listbox" class="LstBox (strict)"() -> ("Item Names"=w318:string[])  [unwired: 2 in, 2 out]
        n127 = for {
          tunnel: w318 -> [w325] mode=indexing
          tunnel: "Action: Update VI Title" ("State") -> [w324]
          tunnel: [w323] -> w316 mode=indexing
          n128 = call <vilib>:"Build State String with Arguments__JKI_lib_State_Machine.vi"("Arguments (\"\")"=w325, "State"=w324) -> ("State with Arguments"=w323:string)  [unwired: 4 in]
        }
        n129 = call "CSM - Compact Multiple States.vi"("Multiple States"=w316) -> ("States"=w315:string)  [unwired: 9 in]
        n130 = call <vilib>:"Add State(s) to Queue__JKI_lib_State_Machine.vi"("State(s) in Front (\"\")"=w315, "State(s) in (\"\")"=w322) -> ("States Out"=w321:string)  [unwired: 13 in]
      }
      frame "Action: Rename Year of copyright" {
        n131 = String To Path(string=w338) -> (path=w339:path)
        n132 = Unbundle By Name(w326) -> ("Root"=w327:path)
        n133 = Build Path(base path=w327, name or relative path=w339) -> (appended path=w337:path)
        n134 = call <vilib>:"Check if File or Folder Exists.vi"("path"=w337) -> ("error out"=w335:errorcluster, "file or folder exists?"=w328:bool, "dup path"=w336:path)  [unwired: 8 in]
        n135 = case shown="True" w328 {
          tunnel: w336 -> [_ w342]
          tunnel: w335 -> [w340 w343]
          tunnel: [w340 w341] -> w333
          frame False {
          }
          frame True {
            n136 = Open VI Reference(vi path=w342, options=2, error in (no error)=w343) -> (vi reference=w346:refnum<vi>, error out=w347:errorcluster)  [unwired: 3 in]
            n137 = call-poly "Is CSM Module.vi"("error in (no error)"=w347, "VIRef"=w346) -> ("error out"=w345:errorcluster, "Is CSM Module?"=w348:bool, "CSM Basic Refs"=w344:T5)  [unwired: 7 in]
            n138 = case shown="True" w348 {
              tunnel: [w352 w365] -> w341
              tunnel: w344 -> [w351 w364]
              tunnel: w345 -> [w353 w363]
              frame False {
                n139 = Unbundle By Name(w351) -> ("VI"=w350:refnum<vi>)
                n140 = Close Reference(reference=w350, error in (no error)=w353) -> (error out=w352:errorcluster)
              }
              frame True {
                n141 = call-poly "CSM-Helper API.vi"("error in (no error)"=w363, "CSM Basic Refs"=w364) -> ("error out"=w360:errorcluster, "CSM-Helper.lvclass"=w361:refnum<class "CSM-Helper.lvclass">)  [unwired: 8 in]
                n142 = Get Date/Time In Seconds() -> (seconds since 1Jan1904=w362:timestamp)
                n143 = disable-structure shown="Disabled" {
                  disable-tunnel: w361 -> [w369 w370]
                  disable-tunnel: w360 -> [w368 w371]
                  disable-tunnel: [w367 w371] -> w359
                  disable-tunnel: [w366 w370] -> w358
                  frame Disabled {
                    n144 = call-poly "CSM-Helper API.vi"("error in (no error)"=w368, "CSM-Helper in"=w369) -> ("error out"=w367:errorcluster, "CSM-Helper out"=w366:refnum<class "CSM-Helper.lvclass">)  [unwired: 8 in]
                  }
                  frame Enabled {
                  }
                }
                n145 = call "Rename Copyright Year.vi"("error in (no error)"=w359, "seconds since 1Jan1904"=w362, "CSM-Helper in"=w358) -> ("error out"=w354:errorcluster, "CSM-Helper out"=w355:refnum<class "CSM-Helper.lvclass">)  [unwired: 7 in]
                n146 = call-poly "CSM-Helper API.vi"("error in (no error)"=w354, "CSM-Helper in"=w355) -> ("error out"=w356:errorcluster, "CSM-Helper out"=w357:refnum<class "CSM-Helper.lvclass">)  [unwired: 8 in]
                n147 = call-poly "CSM-Helper API.vi"("error in (no error)"=w356, "CSM-Helper in"=w357) -> ("error out"=w365:errorcluster)  [unwired: 8 in, 1 out]
              }
            }
          }
        }
        n148 = call <vilib>:"Add State(s) to Queue__JKI_lib_State_Machine.vi"("State(s) in Front (\"\")"="UI: Post Action" ("State(s) in Front (\"\")"), "State(s) in (\"\")"=w330) -> ("States Out"=w331:string)  [unwired: 13 in]
        n149 = Not(x=w333) -> (.not. x?=w332:bool)
        n150 = Bundle By Name(cluster=w326, "Success"=w332) -> (w334:T3)
      }
      frame "Action: Relocate VI Window" {
        w388 = T7 {"Left"=110, "Top"=110, "Right"=0, "Bottom"=0} ("Front Panel Window:Window Bounds")
        w387 = T7 {"Left"=100, "Top"=100, "Right"=0, "Bottom"=0} ("Front Panel Window:Window Bounds")
        n151 = String To Path(string=w407) -> (path=w408:path)
        n152 = Unbundle By Name(w372) -> ("Root"=w373:path)
        n153 = Build Path(base path=w373, name or relative path=w408) -> (appended path=w399:path)
        n154 = Open VI Reference(vi path=w399, options=2) -> (vi reference=w391:refnum<vi>, error out=w394:errorcluster)  [unwired: 4 in]
        n155 = disable-structure shown="Disabled" {
          disable-tunnel: w394 -> [w434 w436]
          disable-tunnel: [w433 w436] -> w393
          disable-tunnel: [w432 w435] -> w392
          disable-tunnel: w391 -> [w431 w435]
          frame Disabled {
            n156 = invoke class="VI" method="FP.Open"(reference=w431, error in=w434) -> (reference out=w432:refnum<vi>, error out=w433:errorcluster)  [unwired: 3 in, 3 out]
          }
          frame Enabled {
          }
        }
        n157 = property class="VI"(reference=w392, error in=w393) -> (reference out=w398:refnum<vi>, error out=w397:errorcluster, "Front Panel.WinBounds"=w390:T7, "BDWin.Bounds"=w389:T7)
        n158 = Unbundle(w387) -> ("Left"=w380:i16, "Top"=w381:i16)  [unwired: 2 out]
        n159 = Unbundle(w389) -> ("Left"=w386:i16, "Top"=w383:i16)  [unwired: 2 out]
        n160 = Unbundle(w388) -> ("Left"=w385:i16, "Top"=w384:i16)  [unwired: 2 out]
        n161 = Unbundle(w390) -> ("Left"=w382:i16, "Top"=w379:i16)  [unwired: 2 out]
        n162 = Not Equal?(x=w379, y=w381) -> (x != y?=w377:bool)
        n163 = Not Equal?(x=w383, y=w384) -> (x != y?=w375:bool)
        n164 = Not Equal?(x=w382, y=w380) -> (x != y?=w378:bool)
        n165 = Not Equal?(x=w386, y=w385) -> (x != y?=w376:bool)
        n166 = Compound Arithmetic op=OR(w378, w377, w376, w375) -> (w374:bool)
        n167 = case shown="False" w374 {
          tunnel: w398 -> [w409 w430]
          tunnel: w397 -> [w410 w429]
          tunnel: [w410 w417] -> w396
          tunnel: [w409 w415] -> w395
          tunnel: w390 -> [_ w414]
          tunnel: w389 -> [_ w413]
          tunnel: w388 -> [_ w412]
          tunnel: w387 -> [_ w411]
          frame False {
          }
          frame True {
            n168 = Subtract(x=w414, y=w411) -> (x-y=w427:T7)
            n169 = Subtract(x=w413, y=w412) -> (x-y=w420:T7)
            n170 = Unbundle(w427) -> ("Left"=w426:i16, "Top"=w425:i16)  [unwired: 2 out]
            n171 = Unbundle(w420) -> ("Left"=w421:i16, "Top"=w422:i16)  [unwired: 2 out]
            n172 = Bundle(cluster=w411, "Left"=w426, "Top"=w425, "Right"=w426, "Bottom"=w425) -> (w424:T7)
            n173 = Bundle(cluster=w412, "Left"=w421, "Top"=w422, "Right"=w421, "Bottom"=w422) -> (w423:T7)
            n174 = Subtract(x=w414, y=w424) -> (x-y=w428:T7)
            n175 = Subtract(x=w413, y=w423) -> (x-y=w419:T7)
            n176 = property class="VI"(reference=w430, error in=w429, "Front Panel.WinBounds"=w428, "BDWin.Bounds"=w419) -> (reference out=w416:refnum<vi>, error out=w418:errorcluster)
            n177 = invoke class="VI" method="Save.Instrument"(reference=w416, error in=w418) -> (reference out=w415:refnum<vi>, error out=w417:errorcluster)  [unwired: 4 in, 4 out]
          }
        }
        n178 = Close Reference(reference=w395, error in (no error)=w396) -> (error out=w405:errorcluster)
        n179 = call <vilib>:"Add State(s) to Queue__JKI_lib_State_Machine.vi"("State(s) in Front (\"\")"="UI: Post Action" ("State(s) in Front (\"\")"), "State(s) in (\"\")"=w402) -> ("States Out"=w403:string)  [unwired: 13 in]
        n180 = Not(x=w405) -> (.not. x?=w404:bool)
        n181 = Bundle By Name(cluster=w372, "Success"=w404) -> (w406:T3)
      }
      frame "Action: Update VI Title" {
        w460 = "(CSM)" ("string")
        n182 = String To Path(string=w445) -> (path=w446:path)
        n183 = Unbundle By Name(w438) -> ("Root"=w439:path)
        n184 = Build Path(base path=w439, name or relative path=w446) -> (appended path=w444:path)
        n185 = Strip Path(path=w444) -> (name=w457:string)  [unwired: 1 out]
        n186 = Open VI Reference(vi path=w444, options=2) -> (vi reference=w466:refnum<vi>, error out=w468:errorcluster)  [unwired: 4 in]
        n187 = Match Pattern(string=w457, regular expression=".vi[m]?$") -> (before substring=w462:string)  [unwired: 1 in, 3 out]
        n188 = property class="VI"(reference=w466, error in=w468) -> (reference out=w465:refnum<vi>, error out=w467:errorcluster, "Front Panel.Title"=w452:string)
        n189 = Match Pattern(string=w452, regular expression=w460) -> (offset past match=w463:i32)  [unwired: 1 in, 3 out]
        n190 = Greater Or Equal To 0?(x=w463) -> ()  [unwired: 1 out]
        n191 = Select(t=w452, s=FALSE, f=w462) -> (s? t:f=w461:string)
        n192 = Search and Replace String(replace all?=TRUE ("replace all? (F)"), input string=w461, search string=w460) -> (result string=w458:string)  [unwired: 5 in, 3 out]
        n193 = call <vilib>:"Trim Whitespace.vi"("string"=w458) -> ("trimmed string"=w456:string)  [unwired: 1 in]
        n194 = Concatenate Strings(w456, " (CSM)" ("string")) -> (w451:string)
        n195 = property class="VI"(reference=w465, error in=w467, "Front Panel.Title"=w451) -> (reference out=w454:refnum<vi>, error out=w453:errorcluster)
        n196 = Not Equal?(x=w452, y=w451) -> (x != y?=w450:bool)
        n197 = Merge Errors(w453) -> (w455:errorcluster)
        n198 = case shown="True" w450 {
          tunnel: [w472 w477] -> w471
          tunnel: [w473 w476] -> w470
          tunnel: w455 -> [w472 w475]
          tunnel: w454 -> [w473 w474]
          frame False {
          }
          frame True {
            n199 = invoke class="VI" method="Save.Instrument"(reference=w474, error in=w475) -> (reference out=w476:refnum<vi>, error out=w477:errorcluster)  [unwired: 4 in, 4 out]
          }
        }
        n200 = Close Reference(reference=w470, error in (no error)=w471) -> (error out=w441:errorcluster)
        n201 = call <vilib>:"Add State(s) to Queue__JKI_lib_State_Machine.vi"("State(s) in Front (\"\")"="UI: Post Action" ("State(s) in Front (\"\")"), "State(s) in (\"\")"=w448) -> ("States Out"=w449:string)  [unwired: 13 in]
        n202 = Bundle("name"=w457, "error out"=w441) -> ()  [unwired: 1 in, 1 out]
        n203 = Not(x=w441) -> (.not. x?=w440:bool)
        n204 = Bundle By Name(cluster=w438, "Success"=w440) -> (w442:T3)
      }
    }
  }
